vi "GetSyncNotifier.vi"(8 "error in (no error)":errorcluster, 11 "SMO in":refnum<class "SMO.lvclass">) -> (0 "error out":errorcluster, 2 "Sync Notifier":refnum<notifier>, 3 "SMO out":refnum<class "SMO.lvclass">)   [LabVIEW 2013, in "SMO.lvclass"]
uses:
  SMO.lvclass
  SMO.lvclass/SMO.ctl
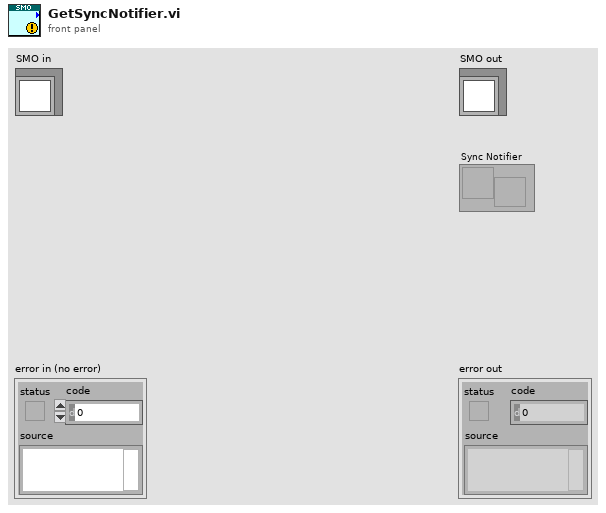
[diagram p1: front panel]
types:
  T1 = typedef "SMO.lvclass/PrivateData--Ref.ctl" = refnum<data-value>
  T2 = typedef "SMO.lvclass/PrivateData--Cluster.ctl" = cluster{"SMO Name":string, "Parent Call":T3, "Registered Processes":T4[], "Sync Notifier":refnum<notifier>, "Process Error Notifier":refnum<notifier>, "Protected Events":T5, "Public Events":T6, "SMO State":T7}
  T3 = typedef "SMO.lvclass/Parent Call--Enum.ctl" = enum16{"Allows parent to run", "Does not request parent to run"}
  T4 = typedef "SMO.lvclass/RegisteredProcessData--Cluster.ctl" = cluster{"Name":string, "Static VI Ref":refnum<vi>, "Running":bool, "NotifierRef":u32}
  T5 = typedef "SMO.lvclass/Protected Events.ctl" = cluster{"StopProcesses":refnum<user-event>, "AbortProcesses":refnum<user-event>}
  T6 = typedef "SMO.lvclass/Public Events.ctl" = cluster{"Error":refnum<user-event>, "State":refnum<user-event>}
  T7 = typedef "SMO.lvclass/SMOState --Enum.ctl" = enum16{"unknown", "Created", "Started", "Stopped"}
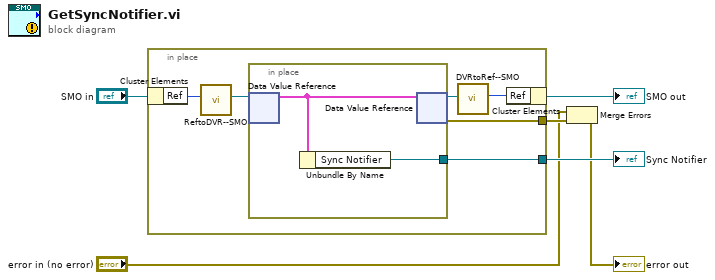
[diagram p0: block diagram]
diagram:
  n1 = in-place {
    in-place-border: [w9] -> w4
    in-place-border: [w8] -> w3
    n2 = in-place-cluster #1("SMO in") -> ("Ref"=w12:u32)
    n3 = call "ReftoDVR--SMO.vi"("Ref"=w12) -> ("Ref"=w10:T1)  [unwired: 10 in]
    n4 = in-place {
      in-place-border: [w13] -> w9
      n5 = in-place-dvr #2(w10) -> (w14:T2)  [unwired: 1 out]
      n6 = Unbundle By Name(w14) -> ("Sync Notifier"=w13:refnum<notifier>)
      n7 = in-place-dvr #2(w14) -> (w7:T1, w8:errorcluster)
    }
    n8 = call "DVRtoRef--SMO.vi"("Ref"=w7) -> ("Ref"=w11:u32)  [unwired: 10 in]
    n9 = in-place-cluster #1("Ref"=w11) -> (→"SMO out":refnum<class "SMO.lvclass">)
  }
  "Sync Notifier" <- w4
  n10 = Merge Errors("error in (no error)", w3) -> (→"error out":errorcluster)
